vi "Read PARTF Root Directory.vi"(8 "error in (no error)":errorcluster, 11 "Config in":refnum<class "Config.lvclass">) -> (0 "error out":errorcluster, 2 "PARTF Root Directory":T1, 3 "Config out":refnum<class "Config.lvclass">)   [LabVIEW 2017, in "Framework.lvlib" / "Config.lvclass"]
uses:
  Config.lvclass
  Typedefs/RootDir.ctl
  Config.lvclass/Config.ctl
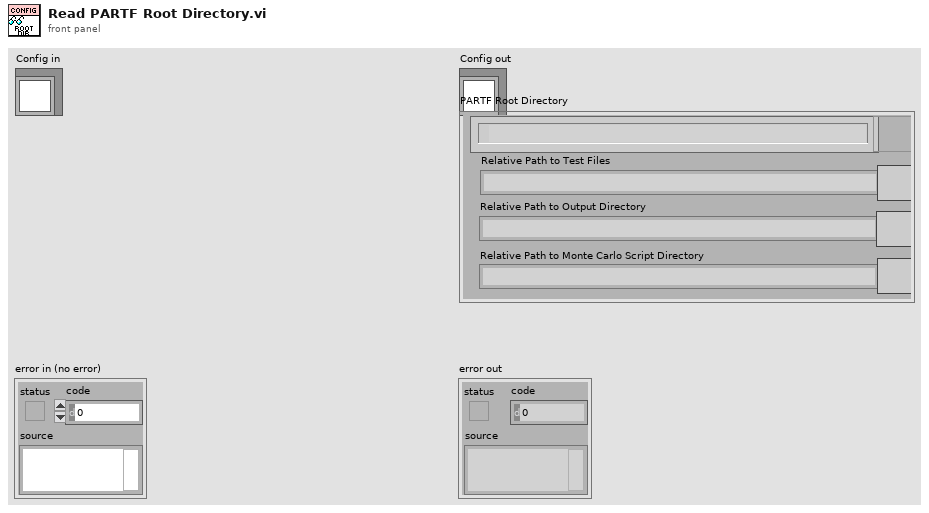
[diagram p1: front panel]
types:
  T1 = typedef "Framework.lvlib/Config.lvclass/RootDir.ctl" = cluster{"pathRootDir":path, "btnOutPath":bool, "OutDir":string, "btnOpenOutputDir":bool, "ScriptDir":string, "btnOpenScriptDir":bool, "TestDir":string, "btnOpenTestDir":bool}
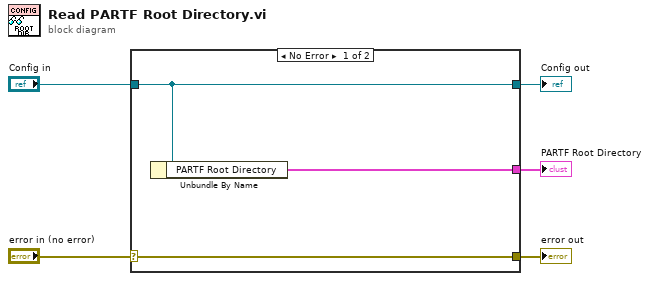
[diagram p0: block diagram]
diagram:
  n1 = case shown="No Error" "error in (no error)" {
    selector: "error in (no error)" -> [w8 w9]
    tunnel: [w8 w9] -> w4
    tunnel: [w7 w10] -> w2
    tunnel: "Config in" -> [w7 w10]
    tunnel: [w6 _] -> w1
    frame No Error {
      n2 = Unbundle By Name(w7) -> ("PARTF Root Directory"=w6:T1)
    }
    frame Error {
    }
  }
  "error out" <- w4
  "Config out" <- w2
  "PARTF Root Directory" <- w1
